vi "Read Network Master.vi"(8 "error in":errorcluster, 11 "Modbus master in":refnum<class "Modbus Master.lvclass">=refnum) -> (0 "error out":errorcluster, 2 "Network Master":refnum<class "Network Master.lvclass">, 3 "Modbus master out":refnum<class "Modbus Master.lvclass">)   [LabVIEW 2021, in "Modbus Master.lvclass"]
doc: "This VI is an accessor for the function definition stored in the Modbus master instance. This accessor can be used as a property node. This function definition is used by the master to determine how to pack and unpack Modbus protocol data units."
uses:
  Modbus Master.lvclass
  API/Modbus API.lvclass
  Network Master.lvclass
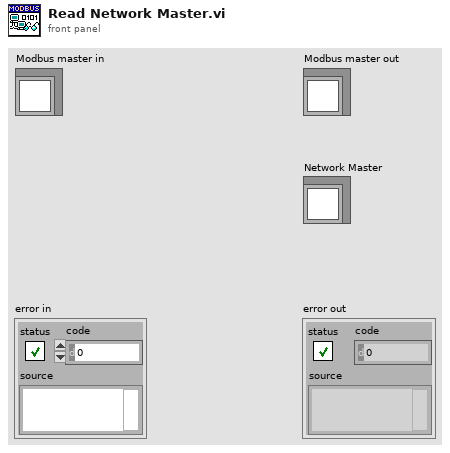
[diagram p1: front panel]
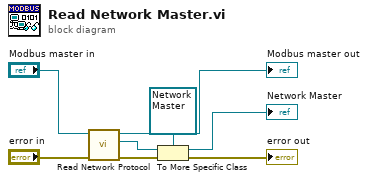
[diagram p0: block diagram]
diagram:
  n1 = call "Read Network Protocol.vi"("error in (no error)"="error in", "Modbus API in"="Modbus master in") -> ("error out"=w5:errorcluster, "Network Protocol"=w6:refnum<class "Network Protocol.lvclass">, "Modbus API out"=→"Modbus master out":refnum<class "Modbus API.lvclass">)  [unwired: 7 in]
  n2 = To More Specific Class(target class=refnum<class "Network Master.lvclass"> refnum ("Network Master"), reference=w6, error in=w5) -> (specific class reference=→"Network Master":refnum<class "Network Master.lvclass">, error out=→"error out":errorcluster)
